vi "String to Version.vi"(11 "String Version":string) -> (3 "Version":T1)   [LabVIEW 2020]
uses:
  Version.ctl
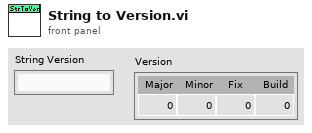
[diagram p1: front panel]
types:
  T1 = typedef "Version.ctl" = cluster{"Major":u16, "Minor":u16, "Fix":u16, "Build":u16}
  T2 = cluster{"[0]":u16, "[1]":u16, "[2]":u16, "[3]":u16}
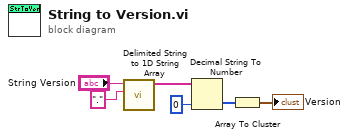
[diagram p0: block diagram]
diagram:
  n1 = call <vilib>:"Delimited String to 1D String Array.vi"("delimiter"=".", "delimited string"="String Version") -> ("string array"=w4:string[])  [unwired: 9 in]
  n2 = Decimal String To Number(string=w4, default (0L)=u16 0 ("default (0 I32)")) -> (number=w2:u16[])  [unwired: 1 in, 1 out]
  n3 = Array To Cluster(array=w2) -> (cluster=→"Version":T2)
